vi "LogSomeData_GaGe4.vi"(0 "Handle Cluster":T1, 1 "tdms file":refnum<k34>, 2 "Save file?":bool, 3 "First chunk?":bool, 5 "Device":T2, 7 "Input settings":T5(array[cluster]), 11 "error in (no error)":errorcluster, 12 "Channel names in":string[](array[string])) -> (6 "Device out":T2, 8 "Input settings out":T5(array[cluster]), 13 "Finished":bool, 14 "Channel names out":string[](array[string]), 15 "error out":errorcluster)   [LabVIEW 2014]
doc: "DESCRIPTION:\nThis VI retrieves the specified amount of data from one or more analog input channels each time a digital start trigger, digital stop trigger, or digital start and stop trigger, occur. It shows how to trigger an acquisition multiple times while avoiding the overhead of configuration and buffer allocation each time. This is a timed acquisition, meaning that a hardware clock is used to control the acquisition rate for fast and accurate timing. It is also a buffered acquisition, meaning that the data are stored in an intermediate memory buffer after they are acquired from the DAQ board. When the pretrigger scans is set to 0, you must set \"choose trigger type\" to START OR STOP TRIGGER (and use a start trigger). Your start trigger will then start your DAQ board and acquisition into a buffer to be read by LabVIEW. When the pretrigger scans is set to greater than 1, you can set \"choose trigger type\" to START OR STOP TRIGGER (and use a stop trigger) or START & STOP TRIGGER (and use both). If you use only the stop trigger, a software strobe starts your DAQ board and your stop trigger will determine when data are acquired into a buffer to be read by LabVIEW. If you use a start and stop trigger, your start trigger will start the DAQ board, but your stop trigger will determine when data are acquired into a buffer to be read by LabVIEW. In either case, your pretrigger scans will be the number of scans to acquire before the stop trigger occurs. The rest of the number of scans to acquire will be after the stop trigger. Data are retrieved from that buffer and displayed after the appropriate amount (before and after the stop trigger) have been acquired. The vertical cursor on the graph indicates where the trigger occurred. With each iteration of the while loop, the VI waits for the next trigger, then reads the same amount of data again from the same channels at the same rate.\n\nUse this VI to wait for multiple digital triggers, acquiring a relatively small amount of data for each trigger (it must fit in the memory available), where each point does not need to be viewed or processed while it is being acquired\n\nINSTRUCTIONS:\n1. Enter the device number, channels, number of scans to acquire, and scan rate.\n2. Enter the pretrigger scans, trigger edge, and time limit.\n3. Set choose trigger type to START OR STOP TRIGGER (to hardware start) if pretrigger scans = 0, If pretrigger scans > 0, set it to START OR STOP TRIGGER (to software start and hardware stop) or START & STOP TRIGGER (to hardware start and hardware stop).\n4. Make the appropriate I/O connections as explained below.\n5. Run the VI.\n\nKEY PARAMETERS:\nThis VI shows how to use the intermediate analog input DAQ VIs to trigger multiple acquisitions. \n\nAI Config.vi is only called on the first iteration of the while loop. This avoids the overhead of configuration and buffer allocation for each acquisition. However, you must stop and restart the VI if you wish to change input parameters.\n\nThe \"read/search mode\" for AI Read.vi is set to \"relative to trigger point\", since this is a hardware triggered acquisition. \n\nAI Control.vi (an advanced analog input VI) is called, in the event that AI Read.vi times out, to momentarily stop the analog input clock. This is needed so the input clock is not running when AI Start.vi (which restarts the clock) is called again.\n\nI/O CONNECTIONS:\nConnect to the input channels on the I/O connector for your board to match the channels you have chosen on the front panel of this VI. For example ACH0 for analog input.\n\nE series boards:\nConnect your start trigger to PFI0/TRIG1, your stop trigger to PFI1/TRIG2.\n\nLegacy MIO boards:\nConnect your start trigger to STARTRIG*, your stop trigger to STOPTRIG.\n\nLegacy MIO-16X, MIO-16F-5, and MIO-64F-5:\nThe start and stop trigger pin is EXTTRIG*.\n\nLab/1200 series boards:\nConnect your start or stop trigger to EXTTRIG. Hardware pretriggering (start & stop) is not supported.\n\nThe PC-LPM-16, DAQCard-500, and DAQCard-700 are not supported by this example.\n\nTo find the actual pin numbers, refer to your hardware user manual.\n\nDAQ VIs USED:\nAI Config.vi, AI Start.vi, AI Read.vi, AI Control.vi, AI Clear.vi."
uses:
  CompuScope LabVIEW SDK/CsLv/CsLV.dll
panel:
  out "Depth":dbl
  out "Segment Size":dbl
  out "Timing out":T3
  in  "Trigger and sampling":T4={"Trig. edge"=enum."Falling", "Trig. source"=enum."External", "Trig. level"=2.0, "Oversample"=FALSE, "Oversamplie by"=1, "Average samples"=TRUE, "Oversample\nto match rates"=FALSE} {"Trig. level" format="%.2f"}
  in  "Timing":T3
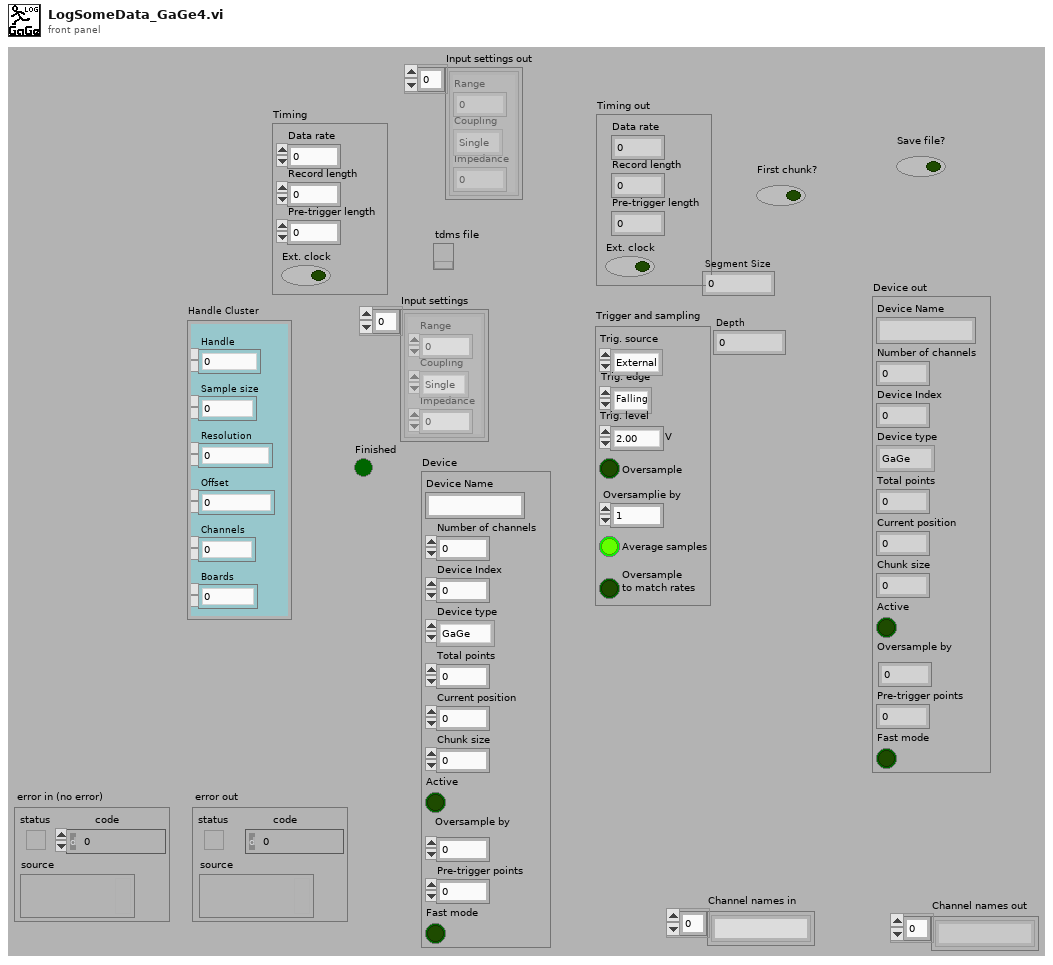
[diagram p1: front panel]
types:
  T1 = cluster{"Handle":u32, "Sample size":u32, "Resolution":i32, "Offset":i32, "Channels":u32, "Boards":u32}
  T2 = cluster{"Device Name":string, "Number of channels":i32, "Device Index":i32, "Device type":enum16{"GaGe", "NI-DAQ", "NI-Scope", "CAMAC", "VXI-1433", "VXI-1437"}, "Total points":i64, "Current position":i64, "Chunk size":i64, "Active":bool, "Oversample by":i32, "Pre-trigger points":i64, "Fast mode":bool}
  T3 = cluster{"Data rate":dbl, "Record length":dbl, "Pre-trigger length":dbl, "Ext. clock":bool}
  T4 = cluster{"Trig. edge":enum16{"Rising", "Falling"}, "Trig. source":enum16{"External", "Immediate"}, "Trig. level":sgl[unit], "Oversample":bool, "Oversamplie by":i32, "Average samples":bool, "Oversample\nto match rates":bool}
  T5 = cluster{"Range":dbl, "Coupling":enum16{"Single", "Differen"}, "Impedance":dbl}[]
  T6 = cluster{"Handle":u32, "Sample Size":u32, "Resolution":i32, "Offset":i32, "Channels":u32, "Boards":u32}
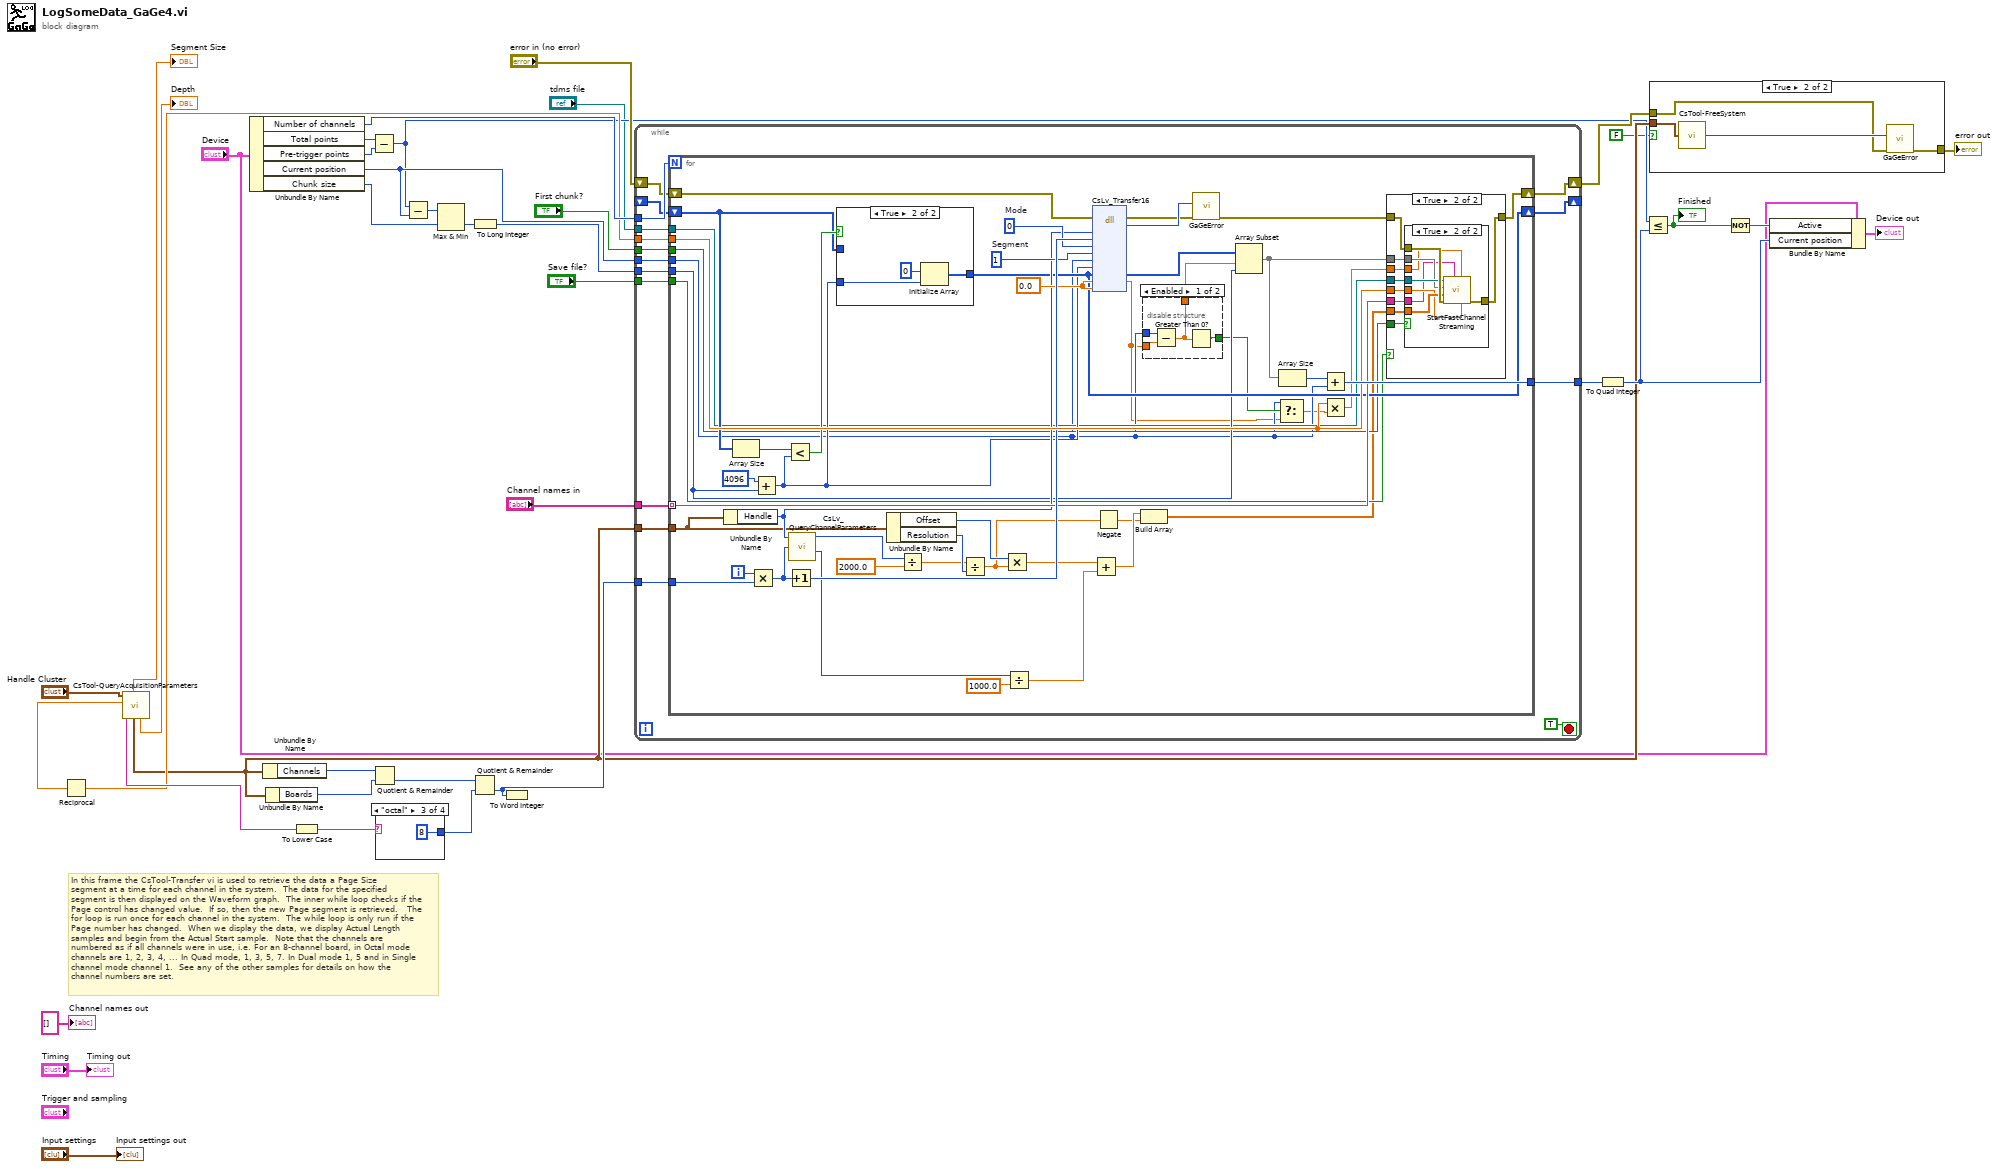
[diagram p0: block diagram]
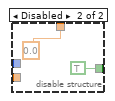
[diagram p2: hidden frame]
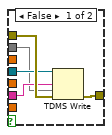
[diagram p4: hidden frame]
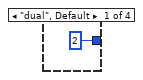
[diagram p6: hidden frame]
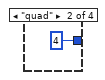
[diagram p7: hidden frame]
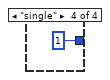
[diagram p8: hidden frame]
diagram:
  # "In this frame the CsTool-Transfer vi is used to retrieve the data a Page Size \nsegment at a time for each channel in the system.  The data for the specified segment is then displayed on the Waveform graph.  The inner while loop checks if the Page control has changed value.  If so, then the new Page segment is retrieved.   The for loop is run once for each channel in the system.  The while loop is only run if the Page number has changed.  When we display the data, we display Actual Length samples and begin from the Actual Start sample.  Note that the channels are numbered as if all channels were in use, i.e. For an 8-channel board, in Octal mode channels are 1, 2, 3, 4, ... In Quad mode, 1, 3, 5, 7. In Dual mode 1, 5 and in Single channel mode channel 1.  See any of the other samples for details on how the channel numbers are set."
  n1 = call "CsTool-QueryAcquisitionParameters.vi"("Handle Cluster"="Handle Cluster") -> ("Depth"=→"Depth":dbl, "Output Handle Cluster"=w15:T6, "Segment Size"=→"Segment Size":dbl, "Mode"=w31:string, "Sample Rate"=w21:dbl)  [unwired: 6 out]
  n2 = Reciprocal(x=w21) -> (1/x=w22:dbl)
  n3 = Unbundle By Name("Device") -> ("Number of channels"=w23:i32, "Total points"=w35:i64, "Pre-trigger points"=w13:i64, "Current position"=w20:i64, "Chunk size"=w24:i64)
  n4 = Unbundle By Name(w15) -> ("Channels"=w26:u32)
  n5 = Unbundle By Name(w15) -> ("Boards"=w29:u32)
  n6 = To Lower Case(string=w31) -> (all lower case string=w30:string)
  n7 = Subtract(x=w35, y=w13) -> (x-y=w14:i64)
  n8 = Quotient & Remainder(x=w26, y=w29) -> (floor(x/y)=w28:u32)  [unwired: 1 out]
  n9 = case shown="\"octal\"" w30 {
    tunnel: [2 4 8 1] -> w27
    frame "dual", Default {
    }
    frame "quad" {
    }
    frame "octal" {
    }
    frame "single" {
    }
  }
  n10 = Subtract(x=w14, y=w20) -> (x-y=w37:i64)
  n11 = Max & Min(x=w37, y=w24) -> (min(x,y)=w38:i64)  [unwired: 1 out]
  n12 = To Long Integer(number=w38) -> (32bit integer=w19:i32)
  n13 = Quotient & Remainder(x=w28, y=w27) -> (floor(x/y)=w25:u32)  [unwired: 1 out]
  n14 = To Word Integer(number=w25) -> ()  [unwired: 1 out]
  n15 = while {
    tunnel: w25 -> [w59]
    tunnel: w23 -> [w58]
    tunnel: w22 -> [w57]
    tunnel: w20 -> [w56]
    tunnel: w19 -> [w55]
    tunnel: [w54] -> w18
    tunnel: w15 -> [w51]
    tunnel: "Channel names in" -> [w50]
    shift-right: [w52] -> w16
    shift-left: "error in (no error)" -> [w53]
    shift-right: [w49] -> _
    shift-left: _ -> [w48]
    tunnel: "tdms file" -> [w46]
    tunnel: "Save file?" -> [w45]
    tunnel: "First chunk?" -> [w44]
    stop <- TRUE stop-if-true
    n16 = for {
      N: w58 -> [_]
      tunnel: w51 -> [w92]
      tunnel: w59 -> [w107]
      tunnel: w57 -> [w105]
      tunnel: w56 -> [w77]
      tunnel: w55 -> [w84]
      tunnel: [w106] -> w54
      shift-right: [w96] -> w52
      shift-left: w53 -> [w83]
      tunnel: w50 -> [w95] mode=indexing
      shift-right: [w89] -> w49
      shift-left: w48 -> [w85]
      tunnel: w45 -> [w80]
      tunnel: w44 -> [w79]
      tunnel: w46 -> [w81]
      i -> [w108]
      w100 = 0.0
      w101 = u32 1  # Segment
      w102 = u32 0  # Mode
      n17 = Unbundle By Name(w92) -> ("Handle"=w94:u32)
      n18 = Array Size(array=w85) -> (size(s)=w86:i32)
      n19 = Multiply(x=w108, y=w107) -> (x*y=w93:u32)
      n20 = Add(x=4096, y=w84) -> (x+y=w87:i32)
      n21 = Less?(x=w86, y=w87) -> (x < y?=w88:bool)
      n22 = Increment(x=w93) -> (x+1=w103:u32)
      n23 = call "CsLv_QueryChannelParameters.vi"("Channel"=w93, "Handle"=w94) -> ("DC Offset (mV)"=w72:i32, "Input Range (mV)"=w71:u32)  [unwired: 5 out]
      n24 = case shown="True" w88 {
        tunnel: w87 -> [_ w141]
        tunnel: [w138 w139] -> w89
        tunnel: w85 -> [w138 _]
        frame False {
        }
        frame True {
          n25 = Initialize Array(i16 0 ("element"), w141) -> (w139:i16[])
        }
      }
      n26 = Unbundle By Name(w92) -> ("Offset"=w68:i32, "Resolution"=w70:i32)
      n27 = Divide(x=w71, y=2000.0) -> (x/y=w69:dbl)
      n28 = Divide(x=w69, y=w70) -> (x/y=w65:dbl)
      n29 = Multiply(x=w68, y=w65) -> (x*y=w67:dbl)
      n30 = Divide(x=w72, y=1000.0) -> (x/y=w66:dbl)
      n31 = dll-call lib="C:/ProjectLocker/NHMFL/LANL/Libraries/GaGe-DAQ/CompuScope LabVIEW SDK/CsLv/CsLV.dll" fn="CsLv_Transfer16"(error in=w83, "Handle"=w94, "Channel"=w103, "Segment"=w102, "Mode"=w101, "Start"=w77, "Length"=w87, "Buffer"=w89, "ActualStart"=w100, "ActualLength"=w100) -> (error out=w82:errorcluster, w99:i32, "Buffer"=w98:i16[], "ActualStart"=w76:dbl)  [unwired: 5 in, 5 out]
      n32 = Add(x=w67, y=w66) -> (x+y=w63:dbl)
      n33 = Negate(x=w65) -> (-x=w62:dbl)
      n34 = Build Array(w63, w62) -> (w64:dbl[])
      n35 = disable-structure shown="Enabled" {
        disable-tunnel: [w112 TRUE] -> w78
        disable-tunnel: w77 -> [w111 _]
        disable-tunnel: w76 -> [w110 _]
        disable-tunnel: [w109 0.0] -> w60
        frame Enabled {
          n36 = Subtract(x=w111, y=w110) -> (x-y=w109:dbl)
          n37 = Greater Than 0?(x=w109) -> (x > 0?=w112:bool)
        }
        frame Disabled {
        }
      }
      n38 = call "GaGeError.vi"("error in (no error)"=w82, "Error Code"=w99) -> ("error out"=w97:errorcluster)  [unwired: 4 in, 5 out]
      n39 = Array Subset(array=w98, index=w60, length=w84) -> (w91:i16[])
      n40 = Select(t=w77, s=w78, f=w76) -> (s? t:f=w75:dbl)
      n41 = Array Size(array=w91) -> (size(s)=w90:i32)
      n42 = Add(x=w90, y=w77) -> (x+y=w106:i64)
      n43 = Multiply(x=w105, y=w75) -> (x*y=w61:dbl)
      n44 = case shown="True" w80 {
        tunnel: [w115 w124] -> w96
        tunnel: w97 -> [w115 w123]
        tunnel: w81 -> [_ w122]
        tunnel: w91 -> [_ w121]
        tunnel: w64 -> [_ w120]
        tunnel: w105 -> [_ w119]
        tunnel: w95 -> [_ w118]
        tunnel: w61 -> [_ w117]
        tunnel: w79 -> [_ w116]
        frame False {
        }
        frame True {
          n45 = case shown="True" w116 {
            tunnel: [w128 w137] -> w124
            tunnel: w123 -> [w129 w136]
            tunnel: w122 -> [w127 w135]
            tunnel: w121 -> [w125 w134]
            tunnel: w120 -> [_ w133]
            tunnel: w119 -> [_ w132]
            tunnel: w118 -> [w126 w131]
            tunnel: w117 -> [_ w130]
            frame False {
              n46 = TDMS Write(0:w127, 7:w126, 9:w125, 11:w129) -> (15:w128:errorcluster)  [unwired: 2 in, 3 out]
            }
            frame True {
              n47 = call "StartFastChannelStreaming.vi"("dt"=w132, "t0"=w130, "channel name(s) in (Untitled)"=w131, "error in (no error)"=w136, "Scaling coefficients"=w133, "Data"=w134, "tdms file"=w135) -> ("error out"=w137:errorcluster)  [unwired: 1 in, 3 out]
            }
          }
        }
      }
    }
  }
  n48 = To Quad Integer(1:w18) -> (0:w32:i64)
  n49 = Less Or Equal?(x=w14, y=w32) -> (x <= y?=w11:bool)
  "Finished" <- w11
  n50 = case shown="True" FALSE {
    tunnel: [w142 w143] -> w39
    tunnel: w16 -> [w142 w144]
    tunnel: w15 -> [_ w146]
    frame False {
    }
    frame True {
      n51 = call "CsTool-FreeSystem.vi"("Handle Cluster"=w146) -> ("Error Code"=w145:i32)
      n52 = call "GaGeError.vi"("error in (no error)"=w144, "Error Code"=w145) -> ("error out"=w143:errorcluster)  [unwired: 4 in, 5 out]
    }
  }
  "error out" <- w39
  n53 = Not(x=w11) -> (.not. x?=w12:bool)
  n54 = Bundle By Name(cluster="Device", "Active"=w12, "Current position"=w32) -> (→"Device out":T2)
  "Input settings out" <- "Input settings"
  "Timing out" <- "Timing"
  "Channel names out" <- string[] [] ("Channel names in")
